vi "Drive Immediate MM.vi"(7 "Description":string, 8 "Command Info In":T1, 10 "Rotational":cluster{"x":dbl}, 11 "Translational":cluster{"x":dbl, "y":dbl}) -> (0 "Command Info Out":T1)   [LabVIEW 2020]
doc: "Often used for joystick control, this VI checks to see that the joystick axes are outside the deadband and updates the motors appropriately."
uses:
  <vilib>/Rock Robotics/WPI/Framework/Command Status Info.ctl
  <vilib>/Rock Robotics/WPI/Framework/Completion Status.ctl
  <vilib>/Rock Robotics/WPI/Framework/Completion Notifier.ctl
  Implementation/Drive Setpoints.ctl
  Implementation/Drive Operations.ctl
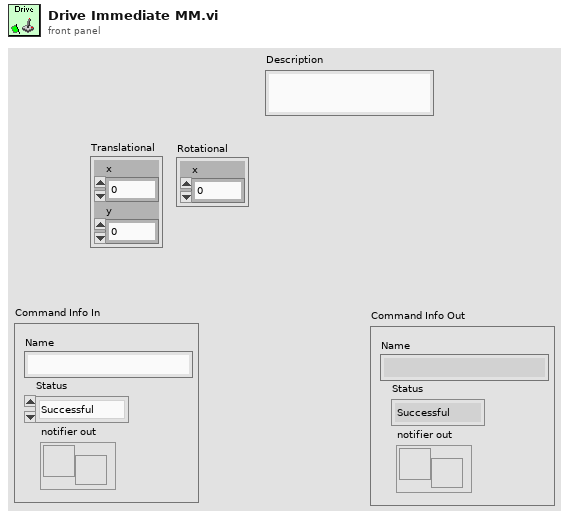
[diagram p1: front panel]
types:
  T1 = typedef "Command Status Info.ctl" = cluster{"Name":string, "Status":T2, "notifier out":T3}
  T2 = typedef "Completion Status.ctl" = enum16{"Successful", "Aborted", "Incomplete"}
  T3 = typedef "Completion Notifier.ctl" = refnum<notifier>
  T4 = typedef "Drive Setpoints.ctl" = cluster{"Operation":T5, "Trans Vel":cluster{"x":dbl, "y":dbl}, "Rot Vel":cluster{"omega":dbl}, "Swerve Path Data":cluster{"Translations":cluster{"x out":dbl, "y out":dbl}[], "Rotations":cluster{"th":dbl}[]}, "reset pods":bool}
  T5 = typedef "Drive Operations.ctl" = enum16{"Reserve", "Read Current", "Immediate", "Calibrate", "Play Path", "Immediate MM"}
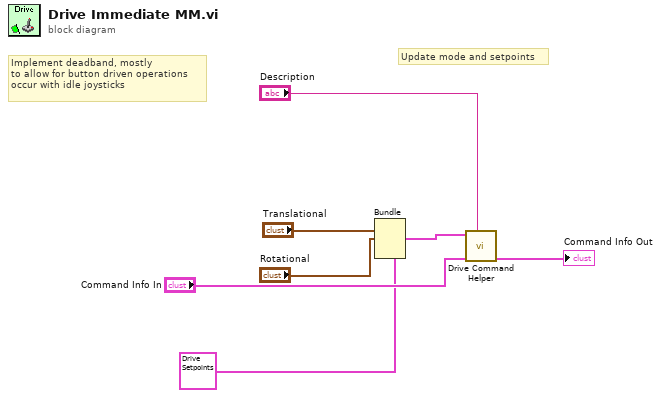
[diagram p0: block diagram]
diagram:
  # "Implement deadband, mostly\nto allow for button driven operations\noccur with idle joysticks"
  # "Update mode and setpoints"
  n1 = Bundle(cluster=T4 {"Operation"=enum."Immediate MM", "Trans Vel"={"x"=0.0, "y"=0.0}, "Rot Vel"={"omega"=0.0}, "Swerve Path Data"={"Translations"=[], "Rotations"=[]}, "reset pods"=FALSE} ("SubSystem Data"), "Trans Vel"="Translational", "Rot Vel"="Rotational") -> (w3:T4)  [unwired: 3 in]
  n2 = call "Drive Command Helper.vi"("Description"="Description", "Command Info In"="Command Info In", "SubSystem Data"=w3) -> ("Command Info Out"=→"Command Info Out":T1)  [unwired: 6 in, 2 out]
